vi "DataCANFileRichInfo.vi"(9 "Language":u32, 11 "file path (dialog if empty)":path caption="文件路径 （空时为对话框）") -> (0 "路径输出":path, 2 "FileInfo":string, 3 "文件类型":string)   [LabVIEW 2015]
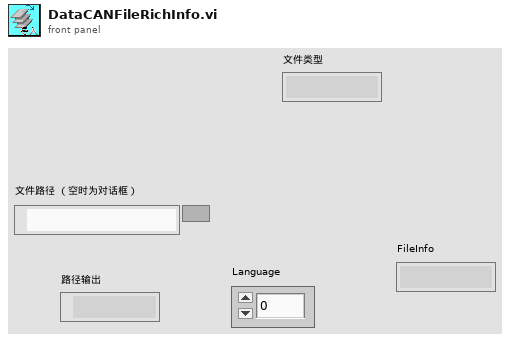
[diagram p1: front panel]
types:
  T1 = enum16{"open", "replace", "create", "open or create", "replace or create", "replace or create with confirmation"}
  T2 = enum16{"big-endian, network order", "native, host order", "little-endian"}
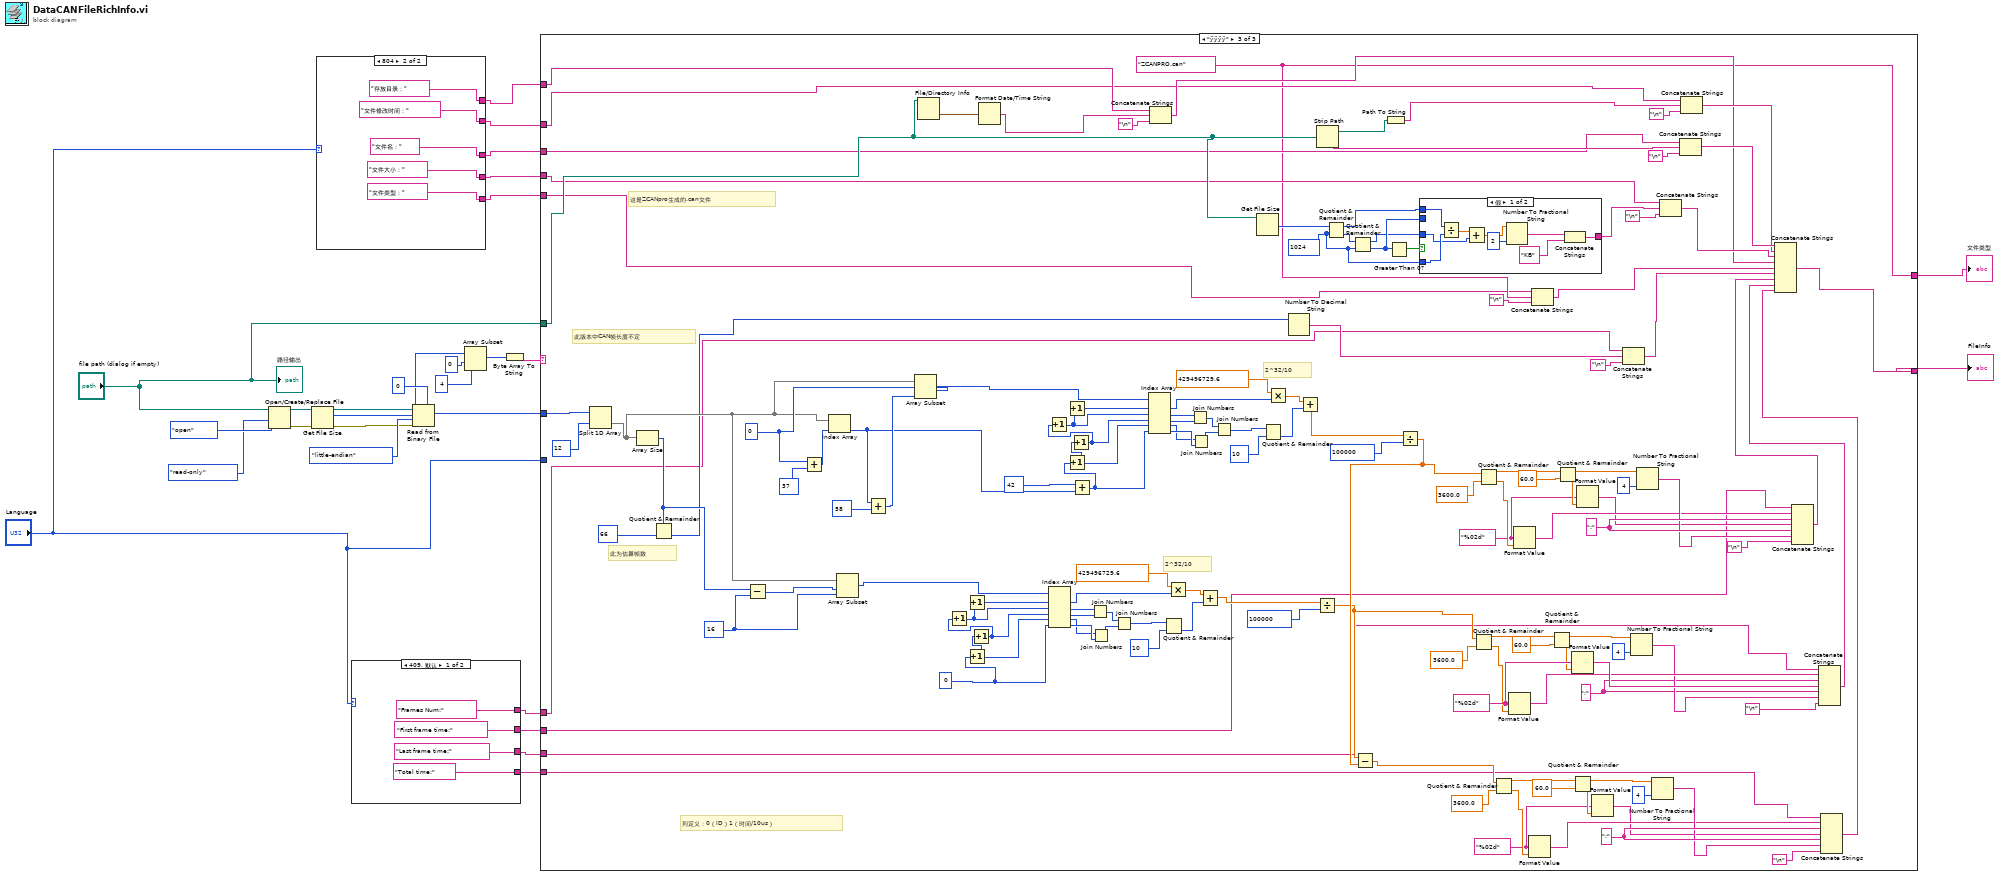
[diagram p0: block diagram]
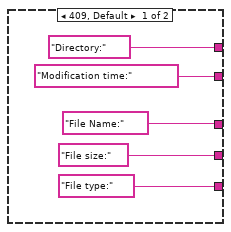
[diagram p2: hidden frame]
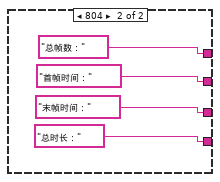
[diagram p3: hidden frame]
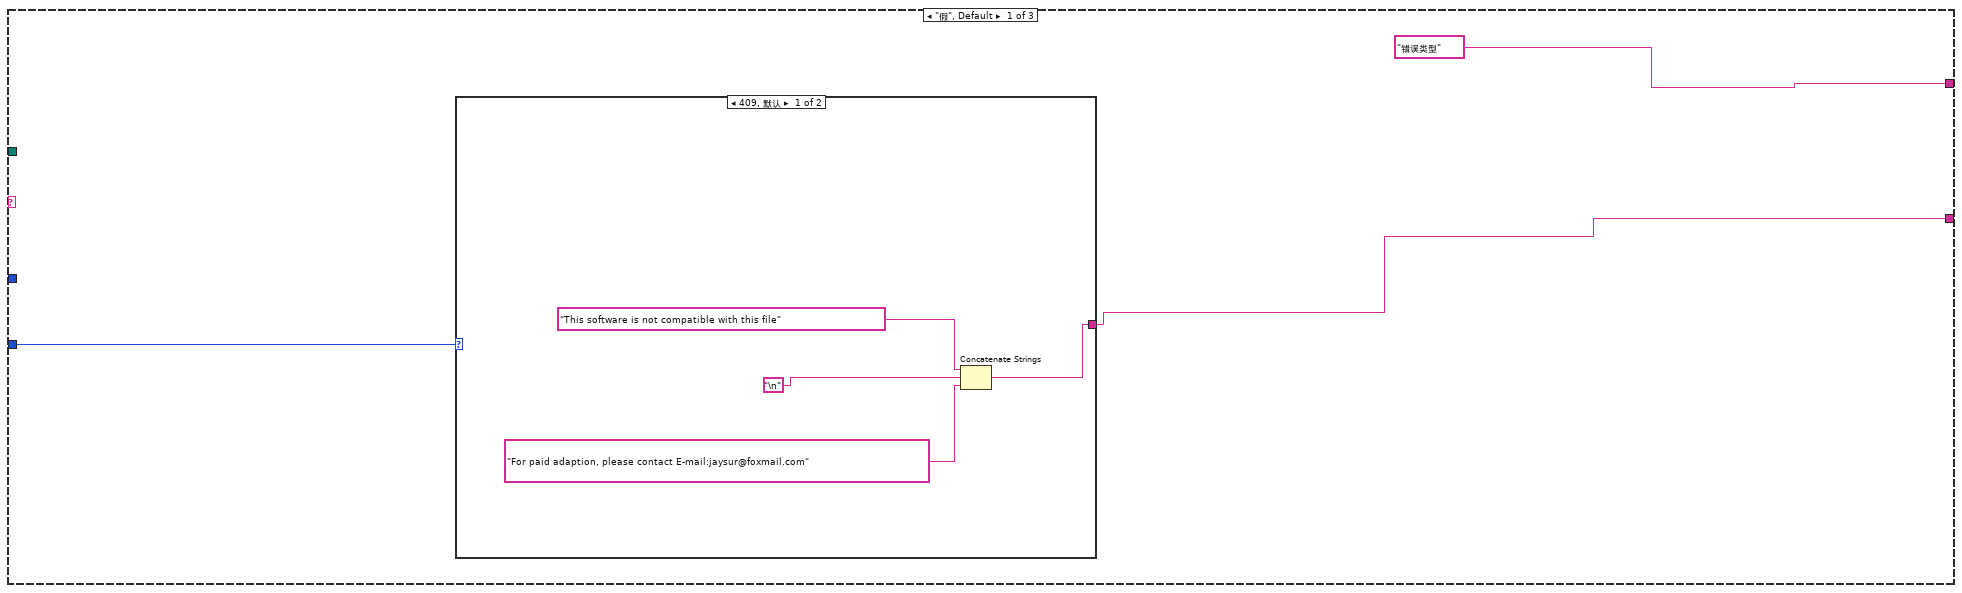
[diagram p4: hidden frame]
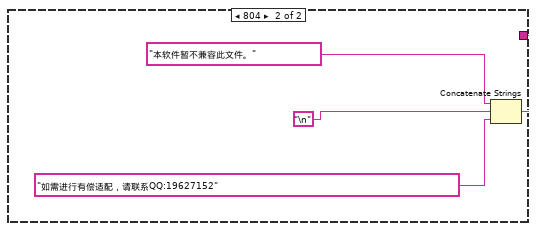
[diagram p5: hidden frame]
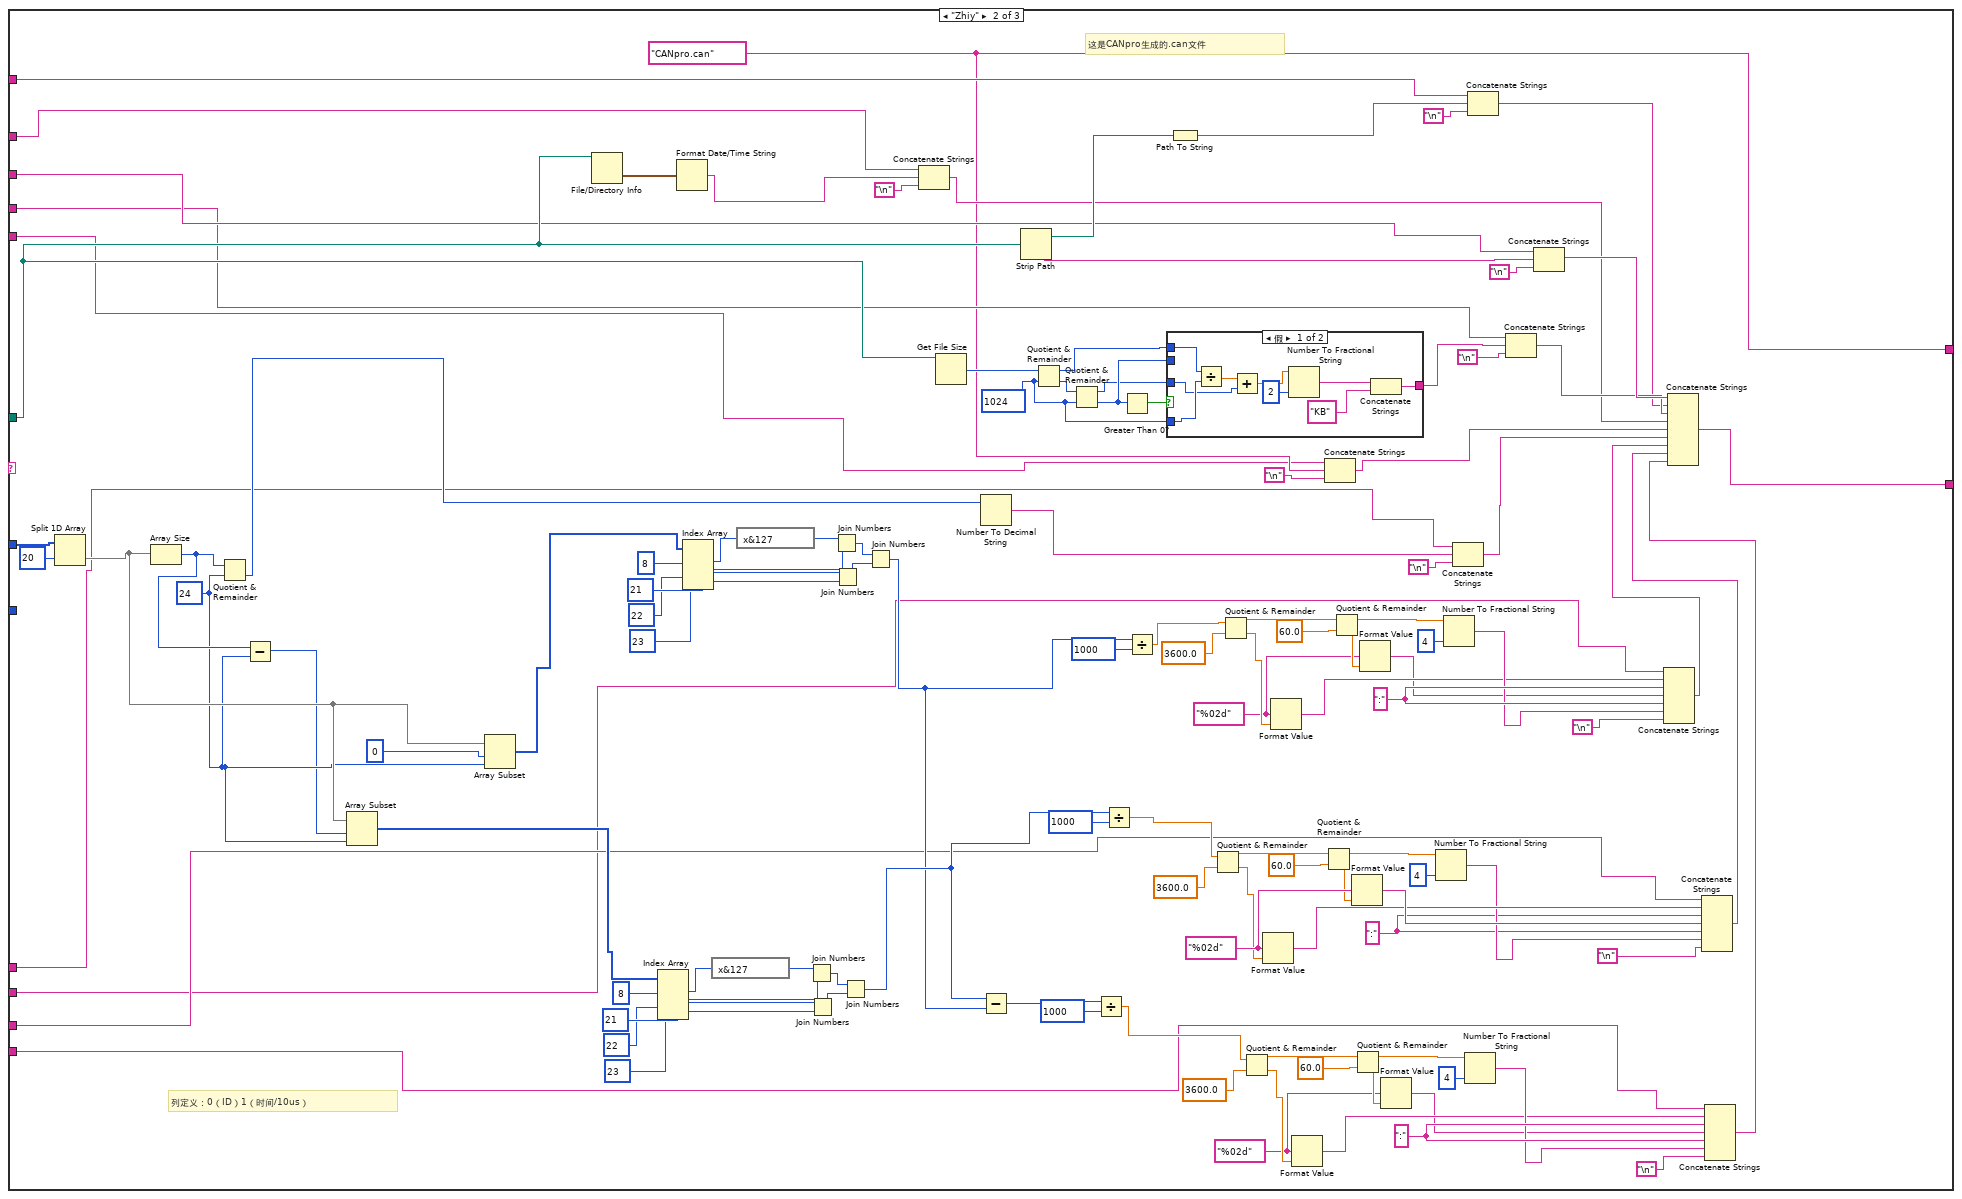
[diagram p6: hidden frame]
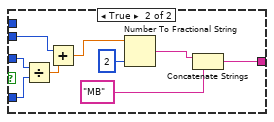
[diagram p7: hidden frame]
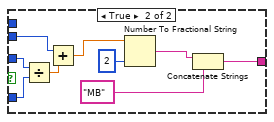
[diagram p8: hidden frame]
diagram:
  n1 = Open/Create/Replace File(file path (use dialog)="file path (dialog if empty)", operation (0:open)=T1."open" ("操作(0:open)"), access (0:read/write)=enum16{"read/write", "read-only", "write-only"}."read-only" ("权限(0:read/write)")) -> (refnum out=w19:refnum<file>, error out=w24:errorcluster)  [unwired: 3 in, 1 out]
  n2 = Get File Size(file=w19, error in=w24) -> (refnum out=w22:refnum<file>, size (in bytes)=w23:i64, 0:w21:errorcluster)
  n3 = case shown="804" "Language" {
    tunnel: ["Modification time:" "文件修改时间："] -> w9
    tunnel: ["Directory:" "存放目录："] -> w8
    tunnel: ["File Name:" "文件名："] -> w7
    tunnel: ["File size:" "文件大小："] -> w6
    tunnel: ["File type:" "文件类型："] -> w5
    frame 409, Default {
    }
    frame 804 {
    }
  }
  n4 = case shown="409, 默认" "Language" {
    tunnel: ["Total time:" "总时长："] -> w4
    tunnel: ["Last frame time:" "末帧时间："] -> w3
    tunnel: ["First frame time:" "首帧时间："] -> w2
    tunnel: ["Frames Num:" "总帧数："] -> w1
    frame 409, Default {
    }
    frame 804 {
    }
  }
  n5 = Read from Binary File(5:u8 0, 8:w21, 9:T2."little-endian" ("字节顺序(0:big-endian, network order)"), 10:w23, 11:w22) -> (2:w15:u8[])  [unwired: 1 in, 3 out]
  n6 = Array Subset(array=w15, index=0 ("索引"), length=4 ("长度")) -> (w16:u8[])
  n7 = Byte Array To String(unsigned byte array=w16) -> (string=w14:string)
  n8 = case shown="\"ÿÿÿÿ\"" w14 {
    tunnel: w15 -> [_ w176 w332]
    tunnel: "file path (dialog if empty)" -> [_ w97 w207]
    tunnel: [w47 w106 w219] -> w12
    tunnel: ["错误类型" w62 w201] -> w11
    tunnel: "Language" -> [w46 _ _]
    tunnel: w9 -> [_ w66 w204]
    tunnel: w8 -> [_ w65 w205]
    tunnel: w7 -> [_ w64 w203]
    tunnel: w6 -> [_ w63 w202]
    tunnel: w5 -> [_ w61 w200]
    tunnel: w4 -> [_ w60 w199]
    tunnel: w3 -> [_ w59 w198]
    tunnel: w2 -> [_ w58 w197]
    tunnel: w1 -> [_ w57 w196]
    frame "假", Default {
      n9 = case shown="409, 默认" w46 {
        tunnel: [w49 w53] -> w47
        frame 409, Default {
          n10 = Concatenate Strings("This software is not compatible with this file", "\n", "For paid adaption, please contact E-mail:jaysur@foxmail.com") -> (w49:string)
        }
        frame 804 {
          n11 = Concatenate Strings("本软件暂不兼容此文件。", "\n", "如需进行有偿适配，请联系QQ:19627152") -> (w53:string)
        }
      }
    }
    frame "Zhiy" {
      w111 = i64 1024 ("y")
      w131 = "%02d" ("格式字符串")
      w137 = ":"
      w154 = "%02d" ("格式字符串")
      w148 = ":"
      w155 = "%02d" ("格式字符串")
      w161 = ":"
      w62 = "CANpro.can"
      w172 = 24 ("y")
      # "列定义：0（ID）1（时间/10us）"
      # "这是CANpro生成的.can文件"
      n12 = Split 1D Array(array=w176, index=20 ("索引")) -> (second subarray=w174:u8[])  [unwired: 1 out]
      n13 = Array Size(array=w174) -> (size(s)=w173:i32)
      n14 = Quotient & Remainder(x=w173, y=w172) -> (floor(x/y)=w105:i32)  [unwired: 1 out]
      n15 = Subtract(x=w173, y=w172) -> (x-y=w169:i32)
      n16 = Array Subset(array=w174, index=w169, length=w172) -> (w81:u8[])
      n17 = Array Subset(array=w174, index=0 ("索引"), length=w172) -> (w68:u8[])
      n18 = File/Directory Info(path=w97) -> (last mod=w96:timestamp)  [unwired: 1 in, 6 out]
      n19 = Index Array(array=w81, index #1=8 ("索引"), index #2=21 ("索引"), index #3=22 ("索引"), index #4=23 ("索引")) -> (element #1=w83:u8, element #2=w86:u8, element #3=w85:u8, element #4=w84:u8)
      n20 = Format Date/Time String(seconds (now)=w96) -> (date/time string=w94:string)  [unwired: 2 in]
      n21 = Index Array(array=w68, index #1=8 ("索引"), index #2=21 ("索引"), index #3=22 ("索引"), index #4=23 ("索引")) -> (element #1=w70:u8, element #2=w73:u8, element #3=w72:u8, element #4=w71:u8)
      n22 = expression code="x&127"(w83) -> (w82:u8)
      n23 = expression code="x&127"(w70) -> (w69:u8)
      n24 = Join Numbers(hi=w82, lo=w86) -> ((hi.lo)=w87:u16)
      n25 = Join Numbers(hi=w85, lo=w84) -> ((hi.lo)=w88:u16)
      n26 = Join Numbers(hi=w69, lo=w73) -> ((hi.lo)=w74:u16)
      n27 = Join Numbers(hi=w72, lo=w71) -> ((hi.lo)=w75:u16)
      n28 = Join Numbers(hi=w87, lo=w88) -> ((hi.lo)=w80:u32)
      n29 = Join Numbers(hi=w74, lo=w75) -> ((hi.lo)=w67:u32)
      n30 = Concatenate Strings(w66, w94, "\n") -> (w93:string)
      n31 = Get File Size(file=w97) -> (size (in bytes)=w114:i64)  [unwired: 1 in, 2 out]
      n32 = Number To Decimal String(number=w105) -> (decimal integer string=w117:string)  [unwired: 1 in]
      n33 = Subtract(x=w80, y=w67) -> (x-y=w167:u32)
      n34 = Strip Path(path=w97) -> (stripped path=w100:path, name=w124:string)
      n35 = Quotient & Remainder(x=w114, y=w111) -> (x-y*floor(x/y)=w107:i64, floor(x/y)=w113:i64)
      n36 = Quotient & Remainder(x=w113, y=w111) -> (x-y*floor(x/y)=w109:i64, floor(x/y)=w110:i64)
      n37 = Divide(x=w167, y=u32 1000) -> (x/y=w127:dbl)
      n38 = Divide(x=w80, y=u32 1000) -> (x/y=w126:dbl)
      n39 = Greater Than 0?(x=w110) -> (x > 0?=w112:bool)
      n40 = Divide(x=w67, y=u32 1000) -> (x/y=w125:dbl)
      n41 = case shown="假" w112 {
        tunnel: w111 -> [w183 w193]
        tunnel: w110 -> [_ w191]
        tunnel: w109 -> [w181 w194]
        tunnel: [w186 w189] -> w108
        tunnel: w107 -> [w184 _]
        frame False {
          n42 = Divide(x=w184, y=w183) -> (x/y=w182:dbl)
          n43 = Add(x=w182, y=w181) -> (x+y=w180:dbl)
          n44 = Number To Fractional String(number=w180, precision (6)=i16 2 ("精度(6)")) -> (F-format string=w178:string)  [unwired: 2 in]
          n45 = Concatenate Strings(w178, "KB" ("字符串")) -> (w186:string)
        }
        frame True {
          n46 = Divide(x=w194, y=w193) -> (x/y=w192:dbl)
          n47 = Add(x=w191, y=w192) -> (x+y=w190:dbl)
          n48 = Number To Fractional String(number=w190, precision (6)=i16 2 ("精度(6)")) -> (F-format string=w188:string)  [unwired: 2 in]
          n49 = Concatenate Strings(w188, "MB") -> (w189:string)
        }
      }
      n50 = Path To String(path=w100) -> (string=w99:string)
      n51 = Quotient & Remainder(x=w126, y=3600.0) -> (x-y*floor(x/y)=w144:dbl, floor(x/y)=w151:dbl)
      n52 = Quotient & Remainder(x=w125, y=3600.0) -> (x-y*floor(x/y)=w165:dbl, floor(x/y)=w158:dbl)
      n53 = Quotient & Remainder(x=w127, y=3600.0) -> (x-y*floor(x/y)=w141:dbl, floor(x/y)=w134:dbl)
      n54 = Format Value(format string=w154, value (0)=w151) -> (output string=w150:string)  [unwired: 1 in]
      n55 = Format Value(format string=w155, value (0)=w158) -> (output string=w159:string)  [unwired: 1 in]
      n56 = Format Value(format string=w131, value (0)=w134) -> (output string=w135:string)  [unwired: 1 in]
      n57 = Quotient & Remainder(x=w144, y=60.0) -> (x-y*floor(x/y)=w146:dbl, floor(x/y)=w152:dbl)
      n58 = Concatenate Strings(w61, w62, "\n") -> (w121:string)
      n59 = Quotient & Remainder(x=w165, y=60.0) -> (x-y*floor(x/y)=w163:dbl, floor(x/y)=w157:dbl)
      n60 = Format Value(format string=w154, value (0)=w152) -> (output string=w153:string)  [unwired: 1 in]
      n61 = Quotient & Remainder(x=w141, y=60.0) -> (x-y*floor(x/y)=w139:dbl, floor(x/y)=w133:dbl)
      n62 = Format Value(format string=w155, value (0)=w157) -> (output string=w156:string)  [unwired: 1 in]
      n63 = Format Value(format string=w131, value (0)=w133) -> (output string=w132:string)  [unwired: 1 in]
      n64 = Number To Fractional String(number=w146, precision (6)=i16 4 ("精度(6)")) -> (F-format string=w149:string)  [unwired: 2 in]
      n65 = Number To Fractional String(number=w163, precision (6)=i16 4 ("精度(6)")) -> (F-format string=w160:string)  [unwired: 2 in]
      n66 = Concatenate Strings(w57, w117, "\n") -> (w118:string)
      n67 = Number To Fractional String(number=w139, precision (6)=i16 4 ("精度(6)")) -> (F-format string=w136:string)  [unwired: 2 in]
      n68 = Concatenate Strings(w65, w99, "\n") -> (w98:string)
      n69 = Concatenate Strings(w63, w108, "\n") -> (w115:string)
      n70 = Concatenate Strings(w64, w124, "\n") -> (w123:string)
      n71 = Concatenate Strings(w58, w159, w161, w156, w161, w160, "\n") -> (w104:string)
      n72 = Concatenate Strings(w59, w150, w148, w153, w148, w149, "\n") -> (w103:string)
      n73 = Concatenate Strings(w60, w135, w137, w132, w137, w136, "\n") -> (w102:string)
      n74 = Concatenate Strings(w123, w98, w115, w93, w121, w118, w104, w103, w102) -> (w106:string)
    }
    frame "ÿÿÿÿ" {
      w224 = i64 1024 ("y")
      w244 = "%02d" ("格式字符串")
      w250 = ":"
      w267 = "%02d" ("格式字符串")
      w261 = ":"
      w268 = "%02d" ("格式字符串")
      w274 = ":"
      w201 = "ZCANPRO.can"
      w285 = 0 ("x+y")
      w304 = 16 ("长度")
      w330 = 0
      # "2^32/10"
      # "2^32/10"
      # "列定义：0（ID）1（时间/10us）"
      # "此为估算帧数"
      # "此版本中CAN帧长度不定"
      # "这是ZCANpro生成的.can文件"
      n75 = Split 1D Array(array=w332, index=12 ("索引")) -> (second subarray=w305:u8[])  [unwired: 1 out]
      n76 = Array Size(array=w305) -> (size(s)=w303:i32)
      n77 = Quotient & Remainder(x=w303, y=66) -> (floor(x/y)=w218:i32)  [unwired: 1 out]
      n78 = Subtract(x=w303, y=w304) -> (x-y=w280:i32)
      n79 = Add(x=w330, y=37) -> (x+y=w316:i32)
      n80 = Index Array(array=w305, index=w316) -> (element=w306:u8)
      n81 = Array Subset(array=w305, index=w280, length=w304) -> (w286:u8[])
      n82 = Add(x=w306, y=u8 58) -> (x+y=w313:u8)
      n83 = Array Subset(array=w305, index=w330, length=w313) -> (w323:u8[])
      n84 = File/Directory Info(path=w207) -> (last mod=w210:timestamp)  [unwired: 1 in, 6 out]
      n85 = Increment(x=w285) -> (x+1=w290:i32)
      n86 = Increment(x=w290) -> (x+1=w289:i32)
      n87 = Increment(x=w289) -> (x+1=w287:i32)
      n88 = Increment(x=w287) -> (x+1=w288:i32)
      n89 = Format Date/Time String(seconds (now)=w210) -> (date/time string=w208:string)  [unwired: 2 in]
      n90 = Index Array(array=w286, index #1=w288, index #2=w287, index #3=w289, index #4=w290, index #5=w285) -> (element #1=w294:u8, element #2=w297:u8, element #3=w298:u8, element #4=w299:u8, element #5=w300:u8)
      n91 = Add(x=42 ("索引"), y=w306) -> (x+y=w311:i32)
      n92 = Increment(x=w311) -> (x+1=w310:i32)
      n93 = Increment(x=w310) -> (x+1=w309:i32)
      n94 = Increment(x=w309) -> (x+1=w307:i32)
      n95 = Increment(x=w307) -> (x+1=w308:i32)
      n96 = Join Numbers(hi=w297, lo=w298) -> ((hi.lo)=w301:u16)
      n97 = Join Numbers(hi=w299, lo=w300) -> ((hi.lo)=w302:u16)
      n98 = Join Numbers(hi=w301, lo=w302) -> ((hi.lo)=w296:u32)
      n99 = Index Array(array=w323, index #1=w308, index #2=w307, index #3=w309, index #4=w310, index #5=w311) -> (element #1=w320:u8, element #2=w324:u8, element #3=w325:u8, element #4=w326:u8, element #5=w327:u8)
      n100 = Concatenate Strings(w205, w208, "\n") -> (w206:string)
      n101 = Quotient & Remainder(x=w296, y=u32 10) -> (floor(x/y)=w291:u32)  [unwired: 1 out]
      n102 = Multiply(x=429496729.6, y=w294) -> (x*y=w292:dbl)
      n103 = Join Numbers(hi=w324, lo=w325) -> ((hi.lo)=w328:u16)
      n104 = Join Numbers(hi=w326, lo=w327) -> ((hi.lo)=w329:u16)
      n105 = Add(x=w292, y=w291) -> (x+y=w282:dbl)
      n106 = Join Numbers(hi=w328, lo=w329) -> ((hi.lo)=w322:u32)
      n107 = Get File Size(file=w207) -> (size (in bytes)=w227:i64)  [unwired: 1 in, 2 out]
      n108 = Quotient & Remainder(x=w322, y=u32 10) -> (floor(x/y)=w317:u32)  [unwired: 1 out]
      n109 = Multiply(x=429496729.6, y=w320) -> (x*y=w318:dbl)
      n110 = Number To Decimal String(number=w218) -> (decimal integer string=w230:string)  [unwired: 1 in]
      n111 = Add(x=w318, y=w317) -> (x+y=w281:dbl)
      n112 = Strip Path(path=w207) -> (stripped path=w213:path, name=w237:string)
      n113 = Divide(x=w282, y=i64 100000) -> (x/y=w240:dbl)
      n114 = Quotient & Remainder(x=w227, y=w224) -> (x-y*floor(x/y)=w220:i64, floor(x/y)=w226:i64)
      n115 = Quotient & Remainder(x=w226, y=w224) -> (x-y*floor(x/y)=w222:i64, floor(x/y)=w223:i64)
      n116 = Path To String(path=w213) -> (string=w212:string)
      n117 = Greater Than 0?(x=w223) -> (x > 0?=w225:bool)
      n118 = Divide(x=w281, y=i64 100000) -> (x/y=w241:dbl)
      n119 = Subtract(x=w240, y=w241) -> (x-y=w239:dbl)
      n120 = case shown="假" w225 {
        tunnel: w224 -> [w339 w349]
        tunnel: w223 -> [_ w347]
        tunnel: w222 -> [w337 w350]
        tunnel: [w342 w345] -> w221
        tunnel: w220 -> [w340 _]
        frame False {
          n121 = Divide(x=w340, y=w339) -> (x/y=w338:dbl)
          n122 = Add(x=w338, y=w337) -> (x+y=w336:dbl)
          n123 = Number To Fractional String(number=w336, precision (6)=i16 2 ("精度(6)")) -> (F-format string=w334:string)  [unwired: 2 in]
          n124 = Concatenate Strings(w334, "KB" ("字符串")) -> (w342:string)
        }
        frame True {
          n125 = Divide(x=w350, y=w349) -> (x/y=w348:dbl)
          n126 = Add(x=w347, y=w348) -> (x+y=w346:dbl)
          n127 = Number To Fractional String(number=w346, precision (6)=i16 2 ("精度(6)")) -> (F-format string=w344:string)  [unwired: 2 in]
          n128 = Concatenate Strings(w344, "MB") -> (w345:string)
        }
      }
      n129 = Quotient & Remainder(x=w240, y=3600.0) -> (x-y*floor(x/y)=w257:dbl, floor(x/y)=w264:dbl)
      n130 = Quotient & Remainder(x=w241, y=3600.0) -> (x-y*floor(x/y)=w278:dbl, floor(x/y)=w271:dbl)
      n131 = Quotient & Remainder(x=w239, y=3600.0) -> (x-y*floor(x/y)=w254:dbl, floor(x/y)=w247:dbl)
      n132 = Format Value(format string=w267, value (0)=w264) -> (output string=w263:string)  [unwired: 1 in]
      n133 = Format Value(format string=w268, value (0)=w271) -> (output string=w272:string)  [unwired: 1 in]
      n134 = Format Value(format string=w244, value (0)=w247) -> (output string=w248:string)  [unwired: 1 in]
      n135 = Concatenate Strings(w200, w201, "\n") -> (w234:string)
      n136 = Quotient & Remainder(x=w257, y=60.0) -> (x-y*floor(x/y)=w259:dbl, floor(x/y)=w265:dbl)
      n137 = Quotient & Remainder(x=w278, y=60.0) -> (x-y*floor(x/y)=w276:dbl, floor(x/y)=w270:dbl)
      n138 = Format Value(format string=w267, value (0)=w265) -> (output string=w266:string)  [unwired: 1 in]
      n139 = Quotient & Remainder(x=w254, y=60.0) -> (x-y*floor(x/y)=w252:dbl, floor(x/y)=w246:dbl)
      n140 = Format Value(format string=w268, value (0)=w270) -> (output string=w269:string)  [unwired: 1 in]
      n141 = Format Value(format string=w244, value (0)=w246) -> (output string=w245:string)  [unwired: 1 in]
      n142 = Concatenate Strings(w196, w230, "\n") -> (w231:string)
      n143 = Number To Fractional String(number=w259, precision (6)=i16 4 ("精度(6)")) -> (F-format string=w262:string)  [unwired: 2 in]
      n144 = Number To Fractional String(number=w276, precision (6)=i16 4 ("精度(6)")) -> (F-format string=w273:string)  [unwired: 2 in]
      n145 = Number To Fractional String(number=w252, precision (6)=i16 4 ("精度(6)")) -> (F-format string=w249:string)  [unwired: 2 in]
      n146 = Concatenate Strings(w202, w221, "\n") -> (w228:string)
      n147 = Concatenate Strings(w203, w237, "\n") -> (w236:string)
      n148 = Concatenate Strings(w204, w212, "\n") -> (w211:string)
      n149 = Concatenate Strings(w197, w272, w274, w269, w274, w273, "\n") -> (w217:string)
      n150 = Concatenate Strings(w198, w263, w261, w266, w261, w262, "\n") -> (w216:string)
      n151 = Concatenate Strings(w199, w248, w250, w245, w250, w249, "\n") -> (w215:string)
      n152 = Concatenate Strings(w236, w211, w228, w206, w234, w231, w217, w216, w215) -> (w219:string)
    }
  }
  "FileInfo" <- w12
  "文件类型" <- w11
  "路径输出" <- "file path (dialog if empty)"
